vi "Clock Initialization.vi"(0 "Boolean in":refnum<vi>, 1 "Output Terminal":tag="/Dev1/PFI2", 5 "Duty Cycle":dbl=0.5 format="%.6f", 7 "Actual Duty Cycle":refnum<vi>, 9 "Frequency":dbl=50.0 format="%.6f", 11 "Actual Frequency":refnum<vi>, 12 "Counter":tag="Dev1/ctr0") -> ()   [LabVIEW 2020]
uses:
  <vilib>/Utility/error.llb/DialogType.ctl
  <vilib>/DAQmx/create/channels.llb/DAQmx Create Channel (CO-Pulse Generation-Frequency).vi
  <vilib>/DAQmx/configure/timing.llb/DAQmx Timing (Implicit).vi
  <resource>/objmgr/daqmx.rc
panel:
  out "Actual Freq":dbl
  out "Actual DutyCyc":dbl
  out "error out":errorcluster
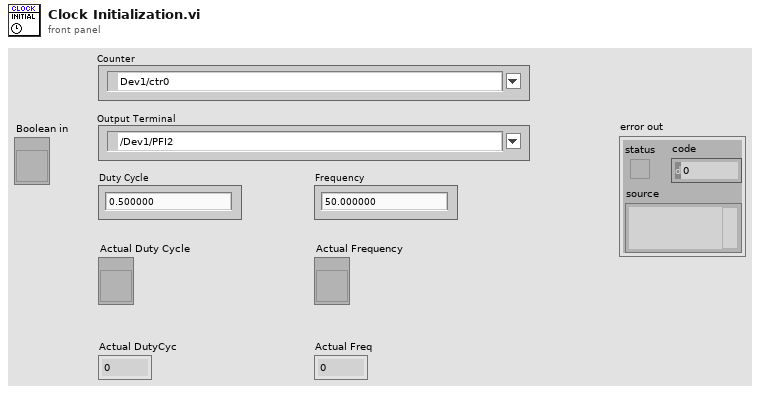
[diagram p1: front panel]
types:
  T1 = typedef "DialogType.ctl" = u16
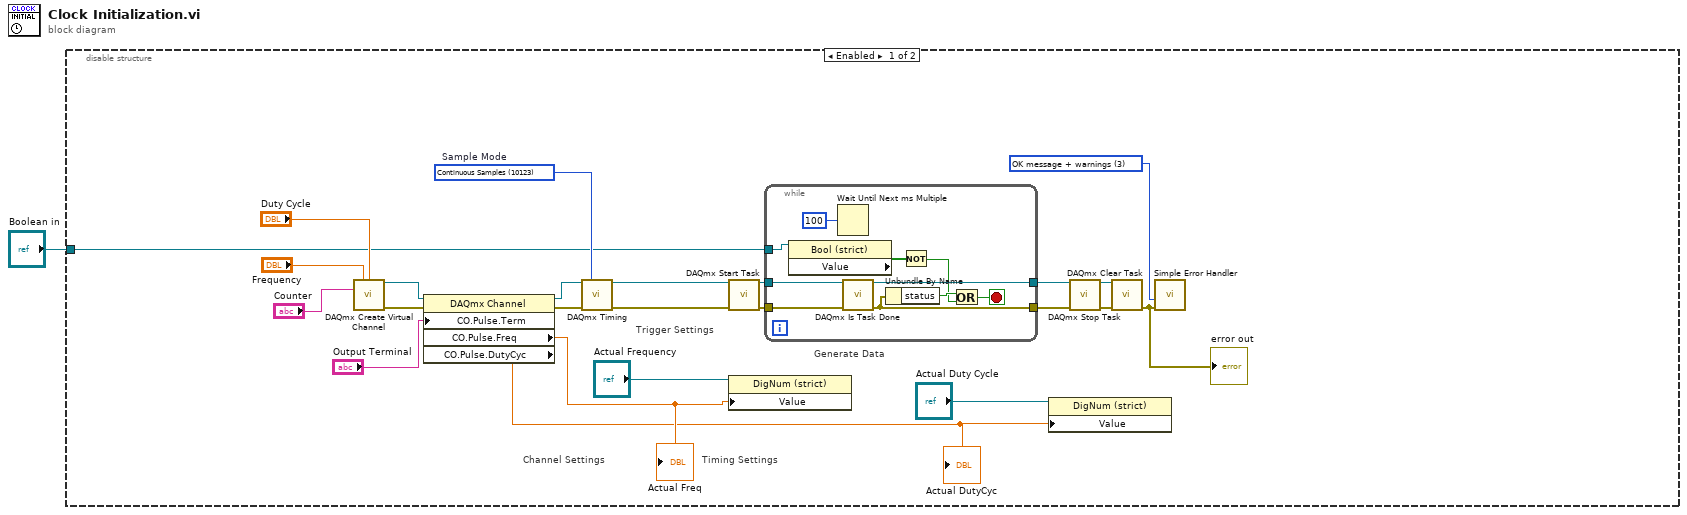
[diagram p0: block diagram]
diagram:
  n1 = disable-structure shown="Enabled" {
    disable-tunnel: "Boolean in" -> [w6 _]
    frame Enabled {
      w9 = T1 3 items=["no dialog", "OK message", "continue or stop message", "OK message + warnings", "continue/stop + warnings"] ("type of dialog (OK msg:1)")
      w25 = 10123 items=["Finite Samples"=10178, "Continuous Samples"=10123, "Hardware Timed Single Point"=12522]  # Sample Mode
      # "Generate Data"
      # "Trigger Settings"
      # "Timing Settings"
      # "Channel Settings"
      n2 = call-poly <vilib>:"DAQmx Create Virtual Channel.vi"("frequency"="Frequency", "duty cycle"="Duty Cycle", "counter"="Counter") -> ("task out"=w20:refnum<k21>, "error out"=w19:errorcluster)  [unwired: 11 in]
      n3 = property class="DAQmx Channel"(reference=w20, error in=w19, "CO.Pulse.Term"="Output Terminal") -> (reference out=w16:refnum<k21>, error out=w17:errorcluster, "CO.Pulse.Freq"=w4:dbl, "CO.Pulse.DutyCyc"=w2:dbl)
      "Actual DutyCyc" <- w2
      "Actual Freq" <- w4
      n4 = call-poly <vilib>:"DAQmx Timing.vi"("task/channels in"=w16, "sample mode"=w25, "error in"=w17) -> ("task out"=w8:refnum<k21>, "error out"=w7:errorcluster)  [unwired: 11 in]
      n5 = call <vilib>:"DAQmx Start Task.vi"("task/channels in"=w8, "error in"=w7) -> ("task out"=w24:refnum<k21>, "error out"=w23:errorcluster)  [unwired: 12 in]
      n6 = property class="DigNum (strict)"(reference="Actual Frequency", "Value"=w4) -> ()  [unwired: 1 in, 2 out]
      n7 = while {
        tunnel: w24 -> [w35]
        tunnel: w23 -> [w34]
        tunnel: [w31] -> w10
        tunnel: [w32] -> w11
        tunnel: w6 -> [w26]
        stop <- w33 stop-if-true
        n8 = property class="Bool (strict)"(reference=w26) -> ("Value"=w27:bool)  [unwired: 1 in, 2 out]
        n9 = Wait Until Next ms Multiple(millisecond multiple=u32 100) -> ()  [unwired: 1 out]
        n10 = call <vilib>:"DAQmx Is Task Done.vi"("task/channels in"=w35, "error in"=w34) -> ("task out"=w32:refnum<k21>, "error out"=w31:errorcluster)  [unwired: 11 in, 1 out]
        n11 = Unbundle By Name(w31) -> ("status"=w30:bool)
        n12 = Not(x=w27) -> (.not. x?=w28:bool)
        n13 = Or(x=w30, y=w28) -> (x .or. y?=w33:bool)
      }
      n14 = property class="DigNum (strict)"(reference="Actual Duty Cycle", "Value"=w2) -> ()  [unwired: 1 in, 2 out]
      n15 = call <vilib>:"DAQmx Stop Task.vi"("task/channels in"=w11, "error in"=w10) -> ("task out"=w13:refnum<k21>, "error out"=w12:errorcluster)  [unwired: 12 in]
      n16 = call <vilib>:"DAQmx Clear Task.vi"("task in"=w13, "error in"=w12) -> ("error out"=w22:errorcluster)  [unwired: 13 in]
      "error out" <- w22
      n17 = call <vilib>:"Simple Error Handler.vi"("type of dialog (OK msg:1)"=w9, "error in (no error)"=w22) -> ()  [unwired: 3 in, 5 out]
    }
    frame Disabled {
    }
  }
